vi "DistanceUpdate.vi"(10 "Delta Time":u32) -> (2 "Disntace":dbl)   [LabVIEW 2016]
uses:
  Globals/Globals.vi
  Globals/InputValues.vi
panel:
  out "Displacement":T1
  out "Linear Acceleration":T2
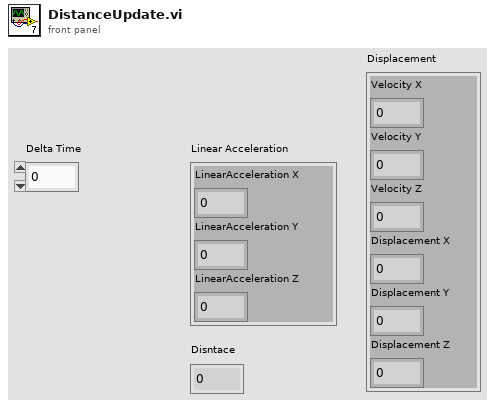
[diagram p1: front panel]
types:
  T1 = cluster{"Velocity X":dbl, "Velocity Y":dbl, "Velocity Z":dbl, "Displacement X":dbl, "Displacement Y":dbl, "Displacement Z":dbl}
  T2 = cluster{"LinearAcceleration X":dbl, "LinearAcceleration Y":dbl, "LinearAcceleration Z":dbl}
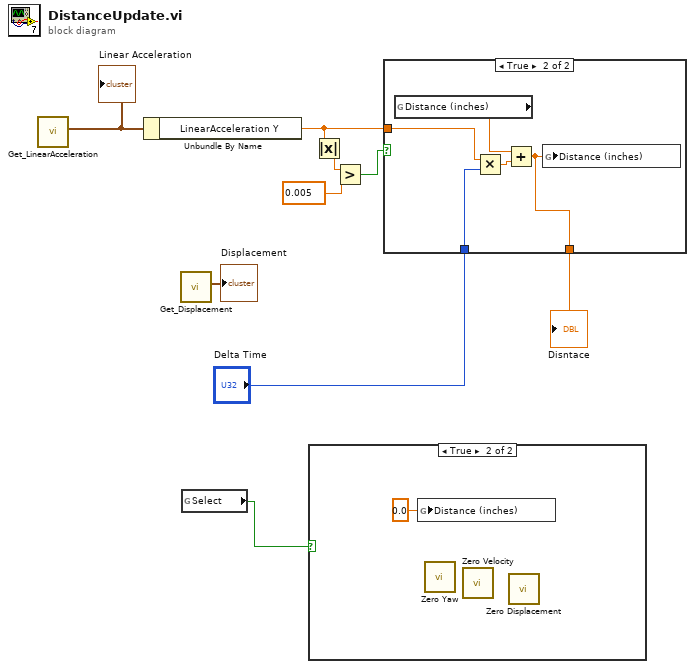
[diagram p0: block diagram]
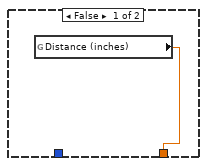
[diagram p3: hidden frame]
diagram:
  n1 = call <vilib>:"Get_LinearAcceleration.vi"() -> ("Linear Acceleration"=w4:T2)  [unwired: 11 in]
  "Linear Acceleration" <- w4
  n2 = Unbundle By Name(w4) -> ("LinearAcceleration Y"=w5:dbl)
  n3 = call <vilib>:"Get_Displacement.vi"() -> ("Displacement"=→"Displacement":T1)  [unwired: 11 in]
  n4 = global read "InputValues.vi" "Select"() -> (w2:bool)
  n5 = case shown="True" w2 {
    frame False {
    }
    frame True {
      n6 = global write "Globals.vi" "Distance (inches)"(0.0 ("Distance (inches)")) -> ()
      n7 = call <vilib>:"Zero Yaw.vi"() -> ()  [unwired: 12 in]
      n8 = call <vilib>:"Zero Velocity.vi"() -> ()  [unwired: 12 in]
      n9 = call <vilib>:"Zero Displacement.vi"() -> ()  [unwired: 12 in]
    }
  }
  n10 = Absolute Value(x=w5) -> (abs(x)=w7:dbl)
  n11 = Greater?(x=w7, y=0.005) -> (0:w8:bool)
  n12 = case shown="True" w8 {
    tunnel: "Delta Time" -> [_ w16]
    tunnel: w5 -> [_ w15]
    tunnel: [w11 w12] -> w9
    frame False {
      n13 = global read "Globals.vi" "Distance (inches)"() -> (w11:dbl)
    }
    frame True {
      n14 = global read "Globals.vi" "Distance (inches)"() -> (w13:dbl)
      n15 = Multiply(x=w15, y=w16) -> (x*y=w14:dbl)
      n16 = Add(x=w13, y=w14) -> (x+y=w12:dbl)
      n17 = global write "Globals.vi" "Distance (inches)"(w12) -> ()
    }
  }
  "Disntace" <- w9
